vi "dataencoder.vi"(7 "Buzz":bool=TRUE, 10 "auto steer":bool=TRUE, 11 "FPGA VI Reference In":refnum<k20>) -> ()   [LabVIEW 2012]
uses:
  RIOGlobal.vi
  <vilib>/Utility/error.llb/Error Cluster From Error Code.vi
  <vilib>/rvi/errors/niLvFpgaAdjustHostInterfaceError.vi
  <vilib>/rvi/interface/nirviReadWriteControl/nirviReadWriteControl.xnode
  NiFpgaLv.dll
  <vilib>/rvi/interface/Simulation/niFpgaSimulationCallBeginRW.vi
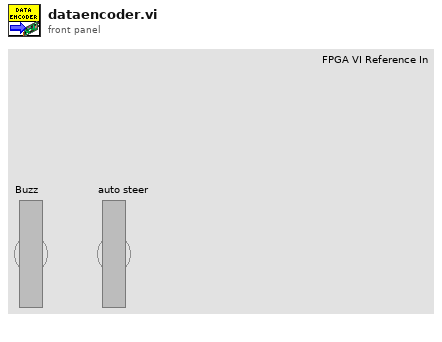
[diagram p1: front panel]
types:
  T1 = cluster{"timestamp high":u32, "timestamp low":u32, "identifier":u32, "type":enum8{"Data Frame", "Remote Frame", "(reserved)", "(reserved) ", "(reserved)  ", "(reserved)   ", "Bus Error", "Transceiver Fault"}, "info A":u8, "info B":u8, "data length":u8, "data":u8[]}
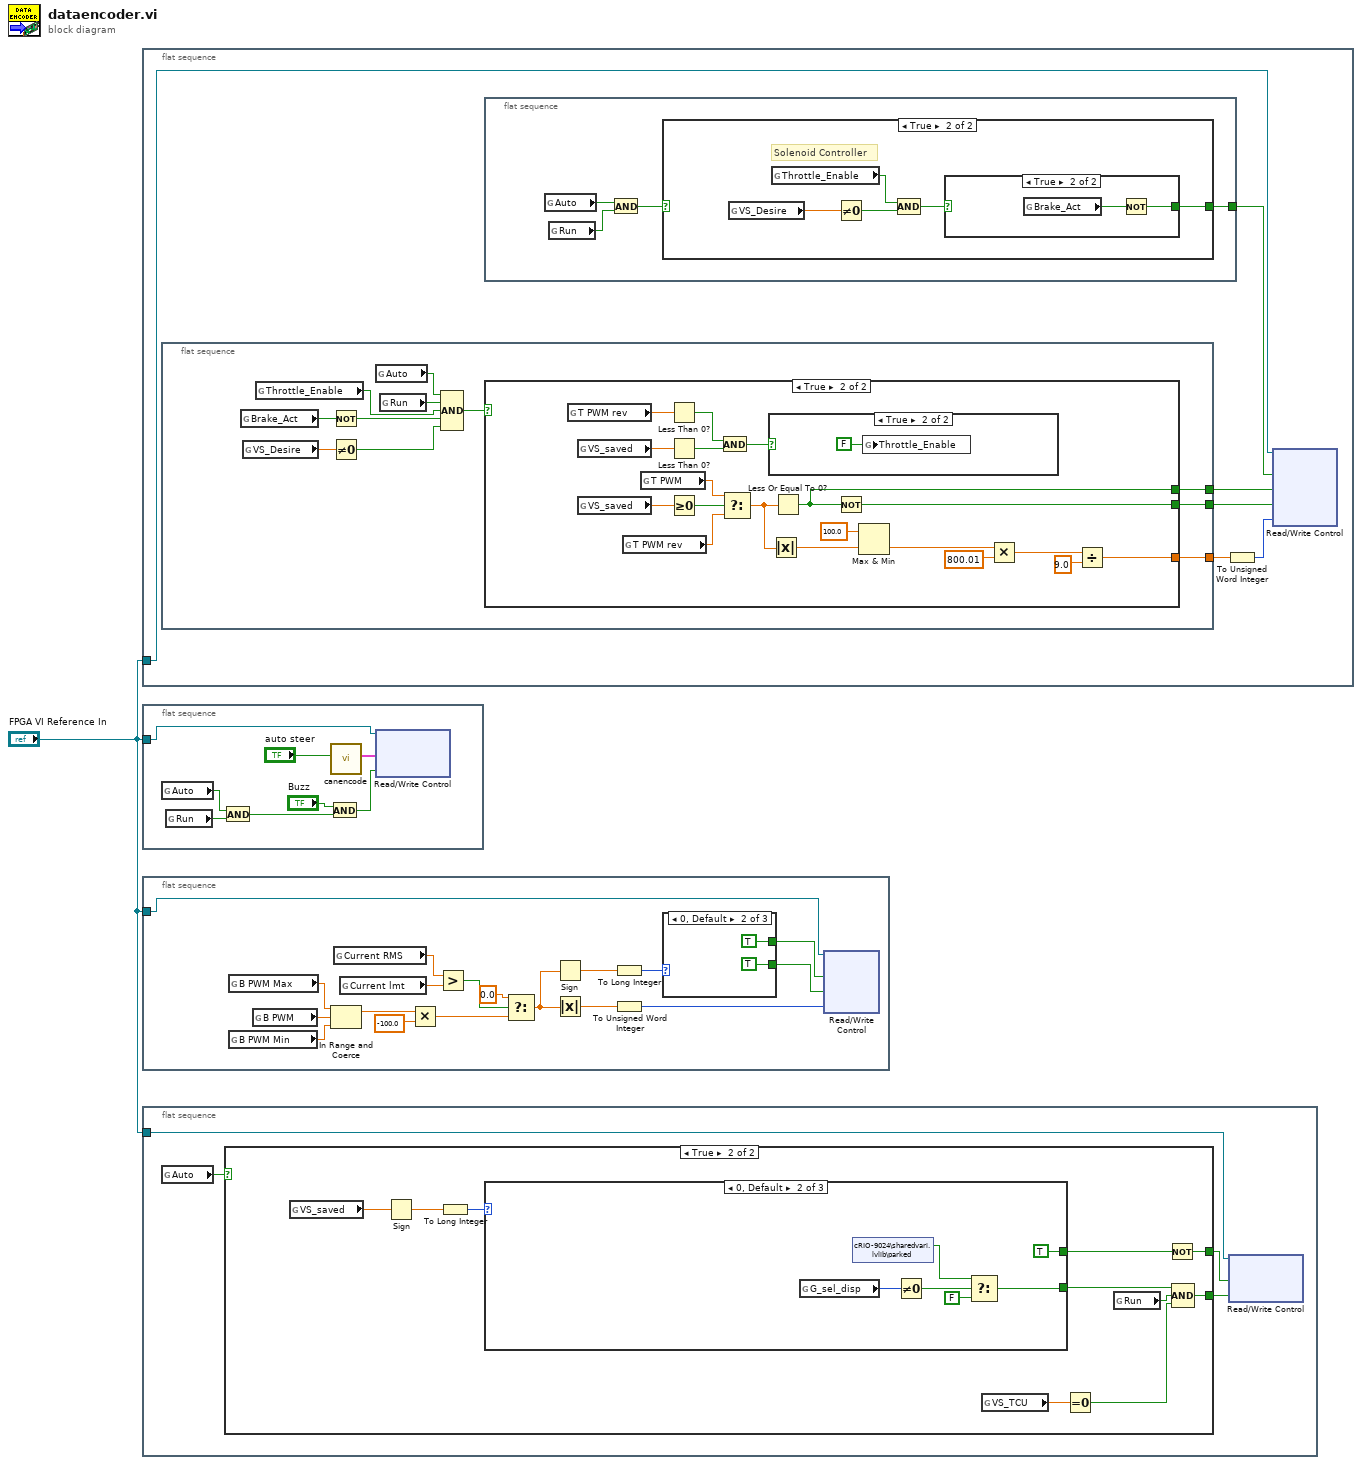
[diagram p0: block diagram]
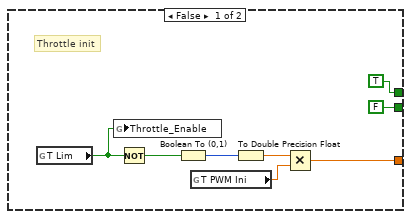
[diagram p4: hidden frame]
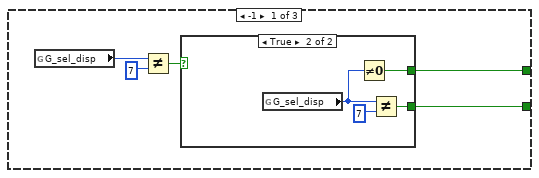
[diagram p7: hidden frame]
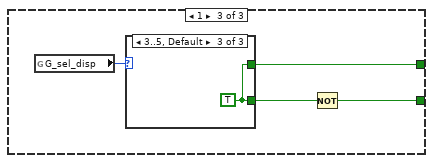
[diagram p9: hidden frame]
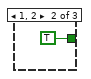
[diagram p11: hidden frame]
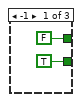
[diagram p12: hidden frame]
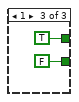
[diagram p13: hidden frame]
diagram:
  n1 = flat-sequence {
    tunnel: "FPGA VI Reference In" -> [w2]
    frame #0 {
      n2 = flat-sequence {
        tunnel: [w30] -> w6
        tunnel: [w29] -> w5
        tunnel: [w28] -> w3
        frame #0 {
          n3 = global read "RIOGlobal.vi" "Brake_Act"() -> (w27:bool)
          n4 = global read "RIOGlobal.vi" "VS_Desire"() -> (w21:dbl)
          n5 = global read "RIOGlobal.vi" "Throttle_Enable"() -> (w26:bool)
          n6 = Not(x=w27) -> (.not. x?=w25:bool)
          n7 = Not Equal To 0?(x=w21) -> (x != 0?=w24:bool)
          n8 = global read "RIOGlobal.vi" "Auto"() -> (w22:bool)
          n9 = global read "RIOGlobal.vi" "Run"() -> (w23:bool)
          n10 = Compound Arithmetic op=AND(w22, w23, w26, w25, w24) -> (w31:bool)
          n11 = case shown="True" w31 {
            tunnel: [TRUE ("T RDir") w56] -> w30
            tunnel: [FALSE ("T Dir") w55] -> w29
            tunnel: [w37 w50] -> w28
            frame False {
              # "Throttle init"
              n12 = global read "RIOGlobal.vi" "T Lim"() -> (w35:bool)
              n13 = global write "RIOGlobal.vi" "Throttle_Enable"(w35) -> ()
              n14 = Not(x=w35) -> (.not. x?=w36:bool)
              n15 = Boolean To (0,1)(Boolean=w36) -> (0, 1=w33:i16)
              n16 = global read "RIOGlobal.vi" "T PWM Ini"() -> (w34:dbl)
              n17 = To Double Precision Float(number=w33) -> (double precision float=w32:dbl)
              n18 = Multiply(x=w32, y=w34) -> (x*y=w37:dbl)
            }
            frame True {
              n19 = global read "RIOGlobal.vi" "T PWM rev"() -> (w40:dbl)
              n20 = global read "RIOGlobal.vi" "VS_saved"() -> (w45:dbl)
              n21 = global read "RIOGlobal.vi" "VS_saved"() -> (w49:dbl)
              n22 = global read "RIOGlobal.vi" "T PWM rev"() -> (w43:dbl)
              n23 = global read "RIOGlobal.vi" "T PWM"() -> (w47:dbl)
              n24 = Less Than 0?(x=w40) -> (x < 0?=w42:bool)
              n25 = Less Than 0?(x=w45) -> (x < 0?=w41:bool)
              n26 = Greater Or Equal To 0?(x=w49) -> (x >= 0?=w48:bool)
              n27 = And(x=w42, y=w41) -> (x .and. y?=w44:bool)
              n28 = Select(t=w47, s=w48, f=w43) -> (s? t:f=w46:dbl)
              n29 = case shown="True" w44 {
                frame False {
                }
                frame True {
                  n30 = global write "RIOGlobal.vi" "Throttle_Enable"(FALSE ("Throttle_Enable")) -> ()
                }
              }
              n31 = Absolute Value(x=w46) -> (abs(x)=w57:dbl)
              n32 = Less Or Equal To 0?(x=w46) -> (x <= 0?=w56:bool)
              n33 = Not(x=w56) -> (.not. x?=w55:bool)
              n34 = Max & Min(x=100.0, y=w57) -> (min(x,y)=w54:dbl)  [unwired: 1 out]
              n35 = Multiply(x=w54, y=800.01) -> (x*y=w52:dbl)
              n36 = Divide(x=w52, y=9.0) -> (x/y=w50:dbl)
            }
          }
        }
      }
      n37 = flat-sequence {
        tunnel: [w11] -> w7
        frame #0 {
          n38 = global read "RIOGlobal.vi" "Auto"() -> (w10:bool)
          n39 = global read "RIOGlobal.vi" "Run"() -> (w9:bool)
          n40 = And(x=w10, y=w9) -> (x .and. y?=w8:bool)
          n41 = case shown="True" w8 {
            selector: w8 -> [w12 _]
            tunnel: [w12 w17] -> w11
            frame False {
              # "Solenoid off"
            }
            frame True {
              # "Solenoid Controller"
              n42 = global read "RIOGlobal.vi" "VS_Desire"() -> (w13:dbl)
              n43 = global read "RIOGlobal.vi" "Throttle_Enable"() -> (w14:bool)
              n44 = Not Equal To 0?(x=w13) -> (x != 0?=w16:bool)
              n45 = Compound Arithmetic op=AND(w14, w16) -> (w15:bool)
              n46 = case shown="True" w15 {
                selector: w15 -> [w18 _]
                tunnel: [w18 w20] -> w17
                frame False {
                }
                frame True {
                  n47 = global read "RIOGlobal.vi" "Brake_Act"() -> (w19:bool)
                  n48 = Not(x=w19) -> (.not. x?=w20:bool)
                }
              }
            }
          }
        }
      }
      n49 = To Unsigned Word Integer(number=w3) -> (unsigned 16bit integer=w4:u16)
      n50 = xnode "Read/Write Control"("FPGA VI Reference In"=w2, "Solenoid"=w7, "T RDir"=w6, "T Dir"=w5, "T Pwm"=w4) -> ()  [unwired: 1 in, 2 out]
    }
  }
  n51 = flat-sequence {
    tunnel: "FPGA VI Reference In" -> [w60]
    frame #0 {
      n52 = global read "RIOGlobal.vi" "Auto"() -> (w64:bool)
      n53 = global read "RIOGlobal.vi" "Run"() -> (w65:bool)
      n54 = And(x=w64, y=w65) -> (x .and. y?=w62:bool)
      n55 = And(x="Buzz", y=w62) -> (x .and. y?=w61:bool)
      n56 = call "canencode.vi"("lock"="auto steer") -> ("CAN Write"=w66:T1)  [unwired: 10 in]
      n57 = xnode "Read/Write Control"("FPGA VI Reference In"=w60, "CAN Write"=w66, "Buzz"=w61) -> ()  [unwired: 1 in, 2 out]
    }
  }
  n58 = flat-sequence {
    tunnel: "FPGA VI Reference In" -> [w73]
    frame #0 {
      n59 = global read "RIOGlobal.vi" "B PWM Max"() -> (w70:dbl)
      n60 = global read "RIOGlobal.vi" "B PWM Min"() -> (w69:dbl)
      n61 = global read "RIOGlobal.vi" "B PWM"() -> (w71:dbl)
      n62 = In Range and Coerce(upper limit=w70, x=w71, lower limit=w69) -> (coerced(x)=w68:dbl)  [unwired: 1 out]
      n63 = global read "RIOGlobal.vi" "Current RMS"() -> (w75:dbl)
      n64 = global read "RIOGlobal.vi" "Current lmt"() -> (w76:dbl)
      n65 = Multiply(x=w68, y=-100.0) -> (x*y=w72:dbl)
      n66 = Greater?(x=w75, y=w76) -> (0:w78:bool)
      n67 = Select(t=0.0, s=w78, f=w72) -> (s? t:f=w74:dbl)
      n68 = Sign(1:w74) -> (0:w83:dbl)
      n69 = Absolute Value(x=w74) -> (abs(x)=w81:dbl)
      n70 = To Long Integer(number=w83) -> (32bit integer=w82:i32)
      n71 = To Unsigned Word Integer(number=w81) -> (unsigned 16bit integer=w79:u16)
      n72 = case shown="0, Default" w82 {
        tunnel: [TRUE TRUE FALSE] -> w84
        tunnel: [FALSE TRUE TRUE] -> w85
        frame -1 {
        }
        frame 0, Default {
        }
        frame 1 {
        }
      }
      n73 = xnode "Read/Write Control"("FPGA VI Reference In"=w73, "B RDir"=w85, "B Dir"=w84, "B Pwm"=w79) -> ()  [unwired: 1 in, 2 out]
    }
  }
  n74 = flat-sequence {
    tunnel: "FPGA VI Reference In" -> [w93]
    frame #0 {
      n75 = global read "RIOGlobal.vi" "Auto"() -> (w94:bool)
      n76 = case shown="True" w94 {
        tunnel: [_ w103] -> w95
        tunnel: [_ w100] -> w92
        frame False {
        }
        frame True {
          n77 = global read "RIOGlobal.vi" "VS_saved"() -> (w105:dbl)
          n78 = Sign(1:w105) -> (0:w99:dbl)
          n79 = To Long Integer(number=w99) -> (32bit integer=w98:i32)
          n80 = case shown="0, Default" w98 {
            tunnel: [w107 w115 w121] -> w102
            tunnel: [w108 TRUE w122] -> w104
            frame -1 {
              n81 = global read "RIOGlobal.vi" "G_sel_disp"() -> (w110:u8)
              n82 = Not Equal?(x=w110, y=u8 7) -> (x != y?=w106:bool)
              n83 = case shown="True" w106 {
                tunnel: [_ w113] -> w108
                tunnel: [_ w111] -> w107
                frame False {
                }
                frame True {
                  n84 = global read "RIOGlobal.vi" "G_sel_disp"() -> (w114:u8)
                  n85 = Not Equal To 0?(x=w114) -> (x != 0?=w113:bool)
                  n86 = Not Equal?(x=w114, y=u8 7) -> (x != y?=w111:bool)
                }
              }
            }
            frame 0, Default {
              n87 = global read "RIOGlobal.vi" "G_sel_disp"() -> (w119:u8)
              n88 = shared-variable "cRIO-9024\\sharedvari.lvlib\\parked"() -> (w117:bool)  [unwired: 1 in, 1 out]
              n89 = Not Equal To 0?(x=w119) -> (x != 0?=w118:bool)
              n90 = Select(t=w117, s=w118, f=FALSE) -> (s? t:f=w115:bool)
            }
            frame 1 {
              n91 = global read "RIOGlobal.vi" "G_sel_disp"() -> (w124:u8)
              n92 = case shown="3..5, Default" w124 {
                tunnel: [_ TRUE ("auto speed") w126] -> w122
                tunnel: [_ _ w126] -> w123
                frame 0, 6, 7 {
                }
                frame 1, 2 {
                }
                frame 3..5, Default {
                  w126 = TRUE
                }
              }
              n93 = Not(x=w123) -> (.not. x?=w121:bool)
            }
          }
          n94 = global read "RIOGlobal.vi" "VS_TCU"() -> (w97:dbl)
          n95 = Equal To 0?(x=w97) -> (x = 0?=w96:bool)
          n96 = global read "RIOGlobal.vi" "Run"() -> (w101:bool)
          n97 = Not(x=w104) -> (.not. x?=w103:bool)
          n98 = Compound Arithmetic op=AND(w102, w101, w96) -> (w100:bool)
        }
      }
      n99 = xnode "Read/Write Control"("FPGA VI Reference In"=w93, "Shift Dir"=w95, "Shift PWM"=w92) -> ()  [unwired: 1 in, 2 out]
    }
  }
